vi "string test_single_cell.vi"(9 "Column":i32, 10 "string":string) -> (3 "String invalid!":bool)   [LabVIEW 2012]
uses:
  <vilib>/regexp/Match Regular Expression.xnode
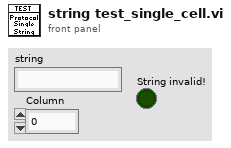
[diagram p1: front panel]
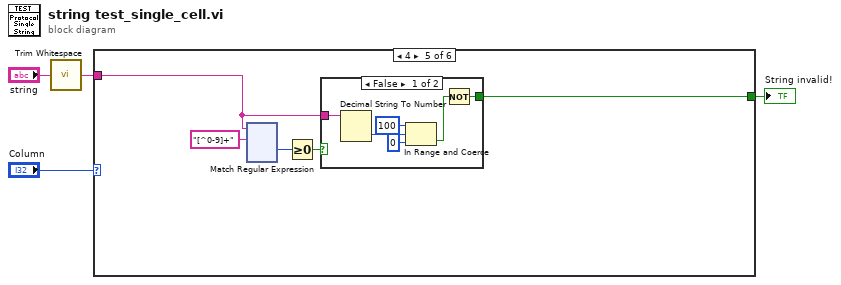
[diagram p0: block diagram]
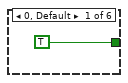
[diagram p2: hidden frame]
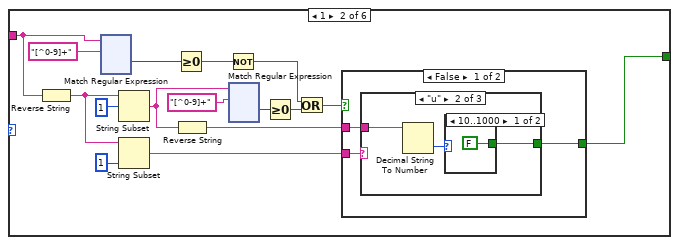
[diagram p3: hidden frame]
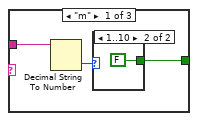
[diagram p4: hidden frame]
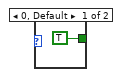
[diagram p5: hidden frame]
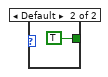
[diagram p6: hidden frame]
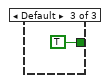
[diagram p7: hidden frame]
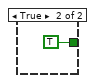
[diagram p8: hidden frame]
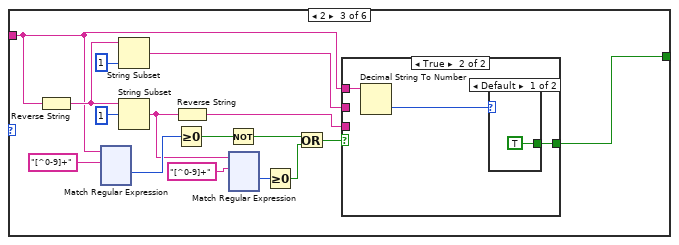
[diagram p9: hidden frame]
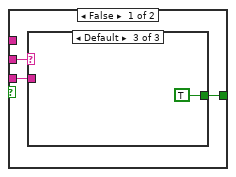
[diagram p10: hidden frame]
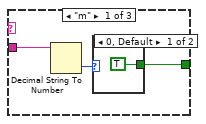
[diagram p11: hidden frame]
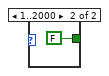
[diagram p12: hidden frame]
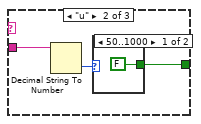
[diagram p13: hidden frame]
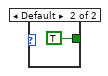
[diagram p14: hidden frame]
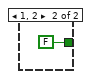
[diagram p15: hidden frame]
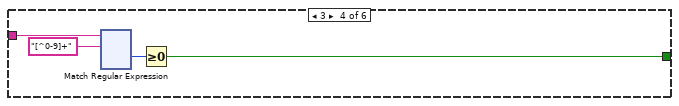
[diagram p16: hidden frame]
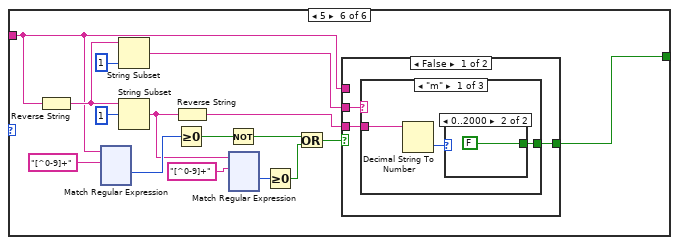
[diagram p18: hidden frame]
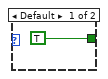
[diagram p19: hidden frame]
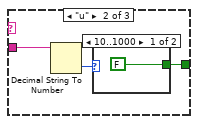
[diagram p20: hidden frame]
diagram:
  n1 = call <vilib>:"Trim Whitespace.vi"("string"="string") -> ("trimmed string"=w4:string)  [unwired: 1 in]
  n2 = case shown="4" "Column" {
    tunnel: w4 -> [_ w16 w259 w517 w632 w754]
    tunnel: [TRUE ("y") w17 w270 w516 w635 w765] -> w1
    frame 0, Default {
    }
    frame 1 {
      n3 = Reverse String(1:w16) -> (0:w14:string)
      n4 = xnode "Match Regular Expression"("input string"=w16, "regular expression"="[^0-9]+") -> ("offset past match"=w21:i32)  [unwired: 4 in, 4 out]
      n5 = String Subset(string=w14, offset (0)=1) -> (substring=w8:string)  [unwired: 1 in]
      n6 = String Subset(string=w14, length (rest)=1 ("length (rest)")) -> (substring=w18:string)  [unwired: 1 in]
      n7 = Greater Or Equal To 0?(x=w21) -> (x >= 0?=w15:bool)
      n8 = Reverse String(1:w8) -> (0:w7:string)
      n9 = Not(x=w15) -> (.not. x?=w9:bool)
      n10 = xnode "Match Regular Expression"("input string"=w8, "regular expression"="[^0-9]+") -> ("offset past match"=w12:i32)  [unwired: 4 in, 4 out]
      n11 = Greater Or Equal To 0?(x=w12) -> (x >= 0?=w10:bool)
      n12 = Or(x=w9, y=w10) -> (x .or. y?=w6:bool)
      n13 = case shown="False" w6 {
        tunnel: w18 -> [w135 _]
        tunnel: [w134 TRUE ("y")] -> w17
        tunnel: w7 -> [w133 _]
        frame False {
          n14 = case shown="\"u\"" w135 {
            tunnel: [w137 w142 TRUE ("y")] -> w134
            tunnel: w133 -> [w136 w141 _]
            frame "m" {
              n15 = Decimal String To Number(string=w136) -> (number=w138:i32)  [unwired: 2 in, 1 out]
              n16 = case shown="1..10" w138 {
                tunnel: [TRUE ("y") FALSE ("y")] -> w137
                frame 0, Default {
                }
                frame 1..10 {
                }
              }
            }
            frame "u" {
              n17 = Decimal String To Number(string=w141) -> (number=w143:i32)  [unwired: 2 in, 1 out]
              n18 = case shown="10..1000" w143 {
                tunnel: [FALSE ("y") TRUE ("y")] -> w142
                frame 10..1000 {
                }
                frame Default {
                }
              }
            }
            frame Default {
            }
          }
        }
        frame True {
        }
      }
    }
    frame 2 {
      n19 = Reverse String(1:w259) -> (0:w268:string)
      n20 = xnode "Match Regular Expression"("input string"=w259, "regular expression"="[^0-9]+") -> ("offset past match"=w274:i32)  [unwired: 4 in, 4 out]
      n21 = String Subset(string=w268, length (rest)=1 ("length (rest)")) -> (substring=w271:string)  [unwired: 1 in]
      n22 = String Subset(string=w268, offset (0)=1) -> (substring=w262:string)  [unwired: 1 in]
      n23 = Greater Or Equal To 0?(x=w274) -> (x >= 0?=w269:bool)
      n24 = Reverse String(1:w262) -> (0:w261:string)
      n25 = Not(x=w269) -> (.not. x?=w263:bool)
      n26 = xnode "Match Regular Expression"("input string"=w262, "regular expression"="[^0-9]+") -> ("offset past match"=w266:i32)  [unwired: 4 in, 4 out]
      n27 = Greater Or Equal To 0?(x=w266) -> (x >= 0?=w264:bool)
      n28 = Or(x=w263, y=w264) -> (x .or. y?=w260:bool)
      n29 = case shown="True" w260 {
        tunnel: w271 -> [w388 _]
        tunnel: [w387 w402] -> w270
        tunnel: w261 -> [w386 _]
        tunnel: w259 -> [_ w401]
        frame False {
          n30 = case shown="Default" w388 {
            tunnel: [w390 w395 TRUE ("y")] -> w387
            tunnel: w386 -> [w389 w394 _]
            frame "m" {
              n31 = Decimal String To Number(string=w389) -> (number=w391:i32)  [unwired: 2 in, 1 out]
              n32 = case shown="0, Default" w391 {
                tunnel: [TRUE ("y") FALSE ("y")] -> w390
                frame 0, Default {
                }
                frame 1..2000 {
                }
              }
            }
            frame "u" {
              n33 = Decimal String To Number(string=w394) -> (number=w396:i32)  [unwired: 2 in, 1 out]
              n34 = case shown="50..1000" w396 {
                tunnel: [FALSE ("y") TRUE ("y")] -> w395
                frame 50..1000 {
                }
                frame Default {
                }
              }
            }
            frame Default {
            }
          }
        }
        frame True {
          n35 = Decimal String To Number(string=w401) -> (number=w400:i32)  [unwired: 2 in, 1 out]
          n36 = case shown="Default" w400 {
            tunnel: [TRUE ("y") FALSE ("y")] -> w402
            frame Default {
            }
            frame 1, 2 {
            }
          }
        }
      }
    }
    frame 3 {
      n37 = xnode "Match Regular Expression"("input string"=w517, "regular expression"="[^0-9]+") -> ("offset past match"=w519:i32)  [unwired: 4 in, 4 out]
      n38 = Greater Or Equal To 0?(x=w519) -> (x >= 0?=w516:bool)
    }
    frame 4 {
      n39 = xnode "Match Regular Expression"("input string"=w632, "regular expression"="[^0-9]+") -> ("offset past match"=w634:i32)  [unwired: 4 in, 4 out]
      n40 = Greater Or Equal To 0?(x=w634) -> (x >= 0?=w631:bool)
      n41 = case shown="False" w631 {
        selector: w631 -> [_ w642]
        tunnel: [w636 w642] -> w635
        tunnel: w632 -> [w638 _]
        frame False {
          n42 = Decimal String To Number(string=w638) -> (number=w641:i32)  [unwired: 2 in, 1 out]
          n43 = In Range and Coerce(upper limit=100, x=w641, lower limit=0) -> (In Range?=w637:bool)  [unwired: 1 out]
          n44 = Not(x=w637) -> (.not. x?=w636:bool)
        }
        frame True {
        }
      }
    }
    frame 5 {
      n45 = Reverse String(1:w754) -> (0:w763:string)
      n46 = xnode "Match Regular Expression"("input string"=w754, "regular expression"="[^0-9]+") -> ("offset past match"=w769:i32)  [unwired: 4 in, 4 out]
      n47 = String Subset(string=w763, length (rest)=1 ("length (rest)")) -> (substring=w766:string)  [unwired: 1 in]
      n48 = String Subset(string=w763, offset (0)=1) -> (substring=w757:string)  [unwired: 1 in]
      n49 = Greater Or Equal To 0?(x=w769) -> (x >= 0?=w764:bool)
      n50 = Reverse String(1:w757) -> (0:w756:string)
      n51 = Not(x=w764) -> (.not. x?=w758:bool)
      n52 = xnode "Match Regular Expression"("input string"=w757, "regular expression"="[^0-9]+") -> ("offset past match"=w761:i32)  [unwired: 4 in, 4 out]
      n53 = Greater Or Equal To 0?(x=w761) -> (x >= 0?=w759:bool)
      n54 = Or(x=w758, y=w759) -> (x .or. y?=w755:bool)
      n55 = case shown="False" w755 {
        tunnel: w766 -> [w883 _]
        tunnel: [w882 w897] -> w765
        tunnel: w756 -> [w881 _]
        tunnel: w754 -> [_ w896]
        frame False {
          n56 = case shown="\"m\"" w883 {
            tunnel: [w885 w890 TRUE ("y")] -> w882
            tunnel: w881 -> [w884 w889 _]
            frame "m" {
              n57 = Decimal String To Number(string=w884) -> (number=w886:i32)  [unwired: 2 in, 1 out]
              n58 = case shown="0..2000" w886 {
                tunnel: [TRUE ("y") FALSE ("y")] -> w885
                frame Default {
                }
                frame 0..2000 {
                }
              }
            }
            frame "u" {
              n59 = Decimal String To Number(string=w889) -> (number=w891:i32)  [unwired: 2 in, 1 out]
              n60 = case shown="10..1000" w891 {
                tunnel: [FALSE ("y") TRUE ("y")] -> w890
                frame 10..1000 {
                }
                frame Default {
                }
              }
            }
            frame Default {
            }
          }
        }
        frame True {
          n61 = Decimal String To Number(string=w896) -> (number=w895:i32)  [unwired: 2 in, 1 out]
          n62 = case shown="1" w895 {
            tunnel: [TRUE ("y") FALSE ("y")] -> w897
            frame Default {
            }
            frame 1 {
            }
          }
        }
      }
    }
  }
  "String invalid!" <- w1
